vi "Update UI User Notification.vi"(4 "Action":enum16{"Reset", "Set", "Initialize"}(ring)=enum."Set", 5 "Progress Bar Value (0)":u8, 6 "Cancel Visibile? (F)":bool, 7 "Progress Bar Visibile? (F)":bool, 8 "Error In":errorcluster, 9 "Busy Cursor? (F)":bool, 10 "Status Bar (\"\")":string, 11 "UI Refs In":T1) -> (0 "Error Out":errorcluster, 3 "UI Refs Out":T1)   [LabVIEW 2015]
uses:
  UI Refs.ctl
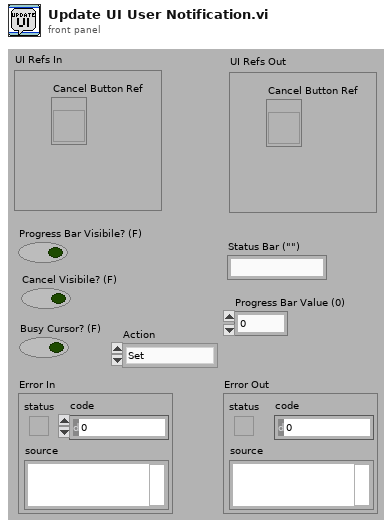
[diagram p1: front panel]
types:
  T1 = typedef "UI Refs.ctl" = cluster{"Cancel Button Ref":refnum<vi>, "Status Bar Text Ref":refnum<vi>, "Progress Bar Ref":refnum<vi>, "This VI":refnum<vi>}
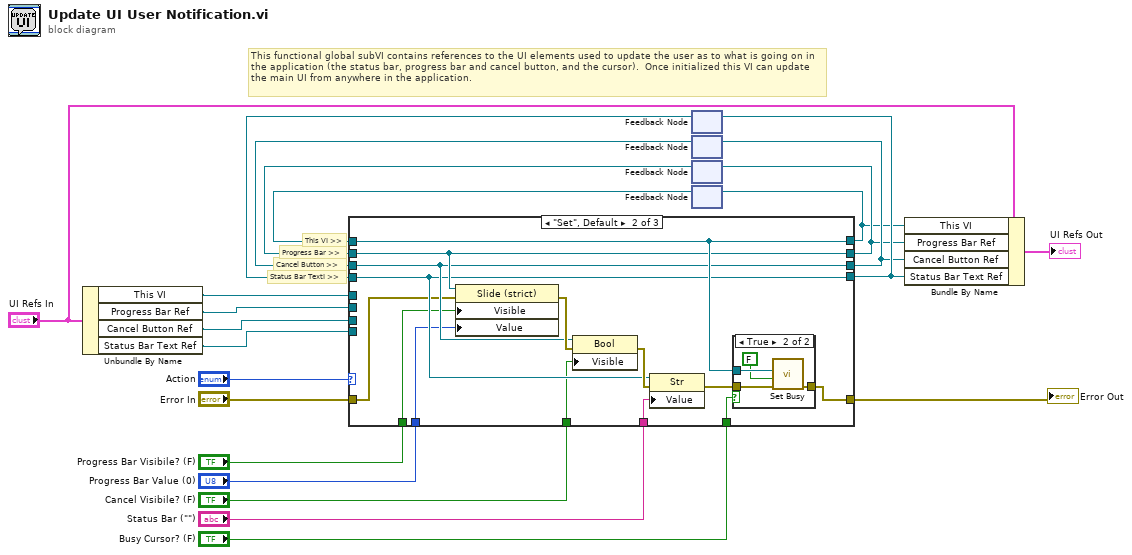
[diagram p0: block diagram]
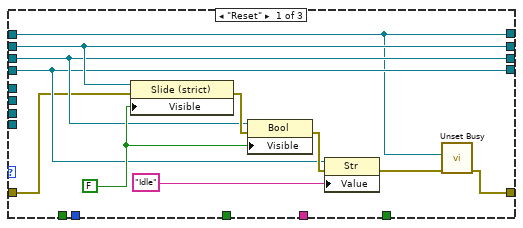
[diagram p2: hidden frame]
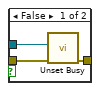
[diagram p3: hidden frame]
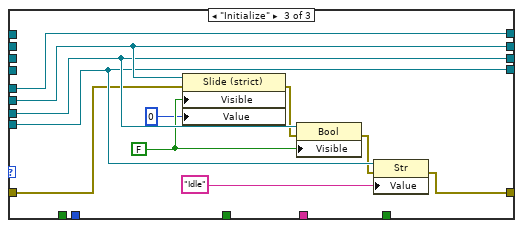
[diagram p4: hidden frame]
diagram:
  # "This functional global subVI contains references to the UI elements used to update the user as to what is going on in the application (the status bar, progress bar and cancel button, and the cursor).  Once initialized this VI can update the main UI from anywhere in the application."
  # "Status Bar TextI >>"
  # "Cancel Button >>"
  # "Progress Bar >>"
  # "This VI >>"
  n1 = Unbundle By Name("UI Refs In") -> ("This VI"=w10:refnum<vi>, "Progress Bar Ref"=w9:refnum<vi>, "Cancel Button Ref"=w8:refnum<vi>, "Status Bar Text Ref"=w7:refnum<vi>)
  n2 = feedback #1() -> (w18:refnum<vi>)  [unwired: 1 in]
  n3 = feedback #2() -> (w19:refnum<vi>)  [unwired: 1 in]
  n4 = feedback #3() -> (w20:refnum<vi>)  [unwired: 1 in]
  n5 = feedback #4() -> (w21:refnum<vi>)  [unwired: 1 in]
  n6 = case shown="\"Set\", Default" "Action" {
    tunnel: w9 -> [_ _ w63]
    tunnel: w8 -> [_ _ w62]
    tunnel: w7 -> [_ _ w61]
    tunnel: w10 -> [_ _ w65]
    tunnel: [w25 w45 w65] -> w1
    tunnel: [w29 w44 w63] -> w2
    tunnel: [w28 w43 w62] -> w3
    tunnel: [w27 w42 w61] -> w4
    tunnel: w21 -> [w25 w45 _]
    tunnel: w20 -> [w29 w44 _]
    tunnel: w19 -> [w28 w43 _]
    tunnel: w18 -> [w27 w42 _]
    tunnel: [w23 w41 w57] -> w16
    tunnel: "Error In" -> [w26 w40 w56]
    tunnel: "Progress Bar Visibile? (F)" -> [_ w38 _]
    tunnel: "Progress Bar Value (0)" -> [_ w37 _]
    tunnel: "Cancel Visibile? (F)" -> [_ w36 _]
    tunnel: "Status Bar (\"\")" -> [_ w35 _]
    tunnel: "Busy Cursor? (F)" -> [_ w34 _]
    frame "Reset" {
      w32 = FALSE ("Visible")
      n7 = property class="Slide (strict)"(reference=w29, error in=w26, "Visible"=w32) -> (error out=w31:errorcluster)  [unwired: 1 out]
      n8 = property class="Bool"(reference=w28, error in=w31, "Visible"=w32) -> (error out=w30:errorcluster)  [unwired: 1 out]
      n9 = property class="Str"(reference=w27, error in=w30, "Value"="Idle" ("Status Bar Text 2")) -> (error out=w24:errorcluster)  [unwired: 1 out]
      n10 = call <vilib>:"Unset Busy.vi"("error in (no error)"=w24, "VI reference (current VI)"=w25) -> ("error out"=w23:errorcluster)  [unwired: 9 in]
    }
    frame "Set", Default {
      n11 = property class="Slide (strict)"(reference=w44, error in=w40, "Visible"=w38, "Value"=w37) -> (error out=w47:errorcluster)  [unwired: 1 out]
      n12 = property class="Bool"(reference=w43, error in=w47, "Visible"=w36) -> (error out=w46:errorcluster)  [unwired: 1 out]
      n13 = property class="Str"(reference=w42, error in=w46, "Value"=w35) -> (error out=w39:errorcluster)  [unwired: 1 out]
      n14 = case shown="True" w34 {
        tunnel: w39 -> [w50 w54]
        tunnel: w45 -> [w49 w53]
        tunnel: [w48 w52] -> w41
        frame False {
          n15 = call <vilib>:"Unset Busy.vi"("error in (no error)"=w50, "VI reference (current VI)"=w49) -> ("error out"=w48:errorcluster)  [unwired: 9 in]
        }
        frame True {
          n16 = call <vilib>:"Set Busy.vi"("error in (no error)"=w54, "disable click? (T)"=FALSE ("Busy?"), "VI reference (current VI)"=w53) -> ("error out"=w52:errorcluster)  [unwired: 7 in, 1 out]
        }
      }
    }
    frame "Initialize" {
      w60 = FALSE ("Visible")
      n17 = property class="Slide (strict)"(reference=w63, error in=w56, "Visible"=w60, "Value"=u8 0) -> (error out=w59:errorcluster)  [unwired: 1 out]
      n18 = property class="Bool"(reference=w62, error in=w59, "Visible"=w60) -> (error out=w58:errorcluster)  [unwired: 1 out]
      n19 = property class="Str"(reference=w61, error in=w58, "Value"="Idle" ("Status Bar Text 2")) -> (error out=w57:errorcluster)  [unwired: 1 out]
    }
  }
  "Error Out" <- w16
  n20 = feedback-in #1(w4) -> ()
  n21 = feedback-in #2(w3) -> ()
  n22 = feedback-in #3(w2) -> ()
  n23 = feedback-in #4(w1) -> ()
  n24 = Bundle By Name(cluster="UI Refs In", "This VI"=w1, "Progress Bar Ref"=w2, "Cancel Button Ref"=w3, "Status Bar Text Ref"=w4) -> (→"UI Refs Out":T1)
